vi "Format Data String.vi"(0 "# pts":dbl, 1 "V_max":dbl, 2 "V_min":dbl, 5 "Linear Scale":bool, 7 "Log Scale":bool, 9 "R_Ref":dbl, 11 "Delay":dbl, 12 "I_Peak":dbl, 13 "I/O Array":dbl[][](array[numeric])) -> (4 "Formatted Data String":string)   [LabVIEW 2020]
doc: "Format Data String.vi outputs a concatenated string of the absolute date and time, headers for data values, and inputted data values in a comma-separated values format."
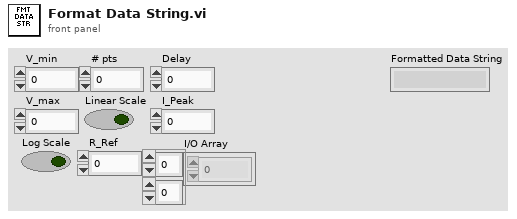
[diagram p1: front panel]
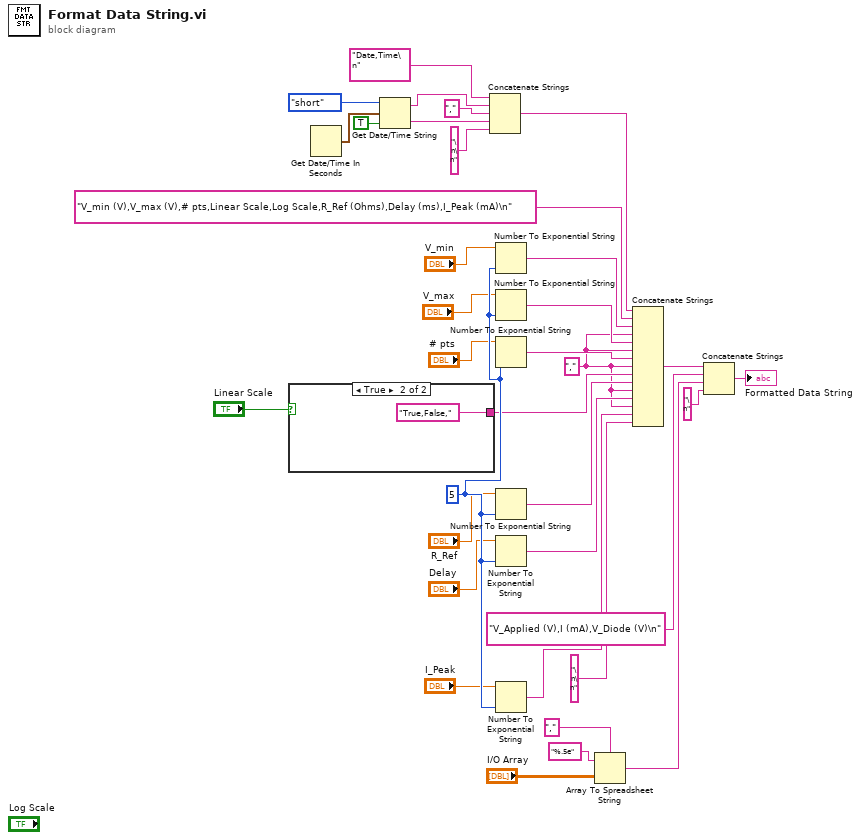
[diagram p0: block diagram]
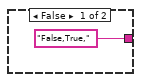
[diagram p2: hidden frame]
diagram:
  w1 = "," ("string")
  w31 = i16 5 ("width (-)")
  n1 = case shown="True" "Linear Scale" {
    tunnel: ["False,True," "True,False,"] -> w26
    frame False {
    }
    frame True {
    }
  }
  n2 = Get Date/Time In Seconds() -> (seconds since 1Jan1904=w19:timestamp)
  n3 = Get Date/Time String(date format (0)=enum16{"short", "long", "abbreviated"}."short", seconds (now)=w19, want seconds? (F)=TRUE) -> (date string=w15:string, time string=w13:string)
  n4 = Concatenate Strings("Date,Time\n" ("string"), w15, "," ("string"), w13, "\n\n" ("string")) -> (w12:string)
  n5 = Number To Exponential String(number="V_min", precision (6)=w31) -> (E-format string=w29:string)  [unwired: 2 in]
  n6 = Number To Exponential String(number="V_max", precision (6)=w31) -> (E-format string=w28:string)  [unwired: 2 in]
  n7 = Number To Exponential String(number="# pts", precision (6)=w31) -> (E-format string=w27:string)  [unwired: 2 in]
  n8 = Number To Exponential String(number="R_Ref", precision (6)=w31) -> (E-format string=w25:string)  [unwired: 2 in]
  n9 = Number To Exponential String(number="Delay", precision (6)=w31) -> (E-format string=w24:string)  [unwired: 2 in]
  n10 = Number To Exponential String(number="I_Peak", precision (6)=w31) -> (E-format string=w23:string)  [unwired: 2 in]
  n11 = Array To Spreadsheet String(delimiter (Tab)=",", array="I/O Array", 3:"%.5e" ("format string")) -> (spreadsheet string=w32:string)
  n12 = Concatenate Strings(w12, "V_min (V),V_max (V),# pts,Linear Scale,Log Scale,R_Ref (Ohms),Delay (ms),I_Peak (mA)\n" ("string"), w29, w1, w28, w1, w27, w1, w26, w25, w1, w24, w1, w23, "\n\n" ("string")) -> (w21:string)
  n13 = Concatenate Strings(w21, "V_Applied (V),I (mA),V_Diode (V)\n" ("string"), w32, "\n" ("string")) -> (→"Formatted Data String":string)
